vi "SetStart_popup.vi"(0 "Input Line Command":string, 3 "error in (no error)":errorcluster, 5 "Delta Trigger":string, 7 "Trigger":string) -> (8 "Output Line Command":string, 9 "Cancel":bool, 10 "error out":errorcluster)   [LabVIEW 2019]
panel:
  in  "platform":u16(ring) items=["Mac", "PC"]
  in  "Cancel button":bool
  in  "OK Button":bool
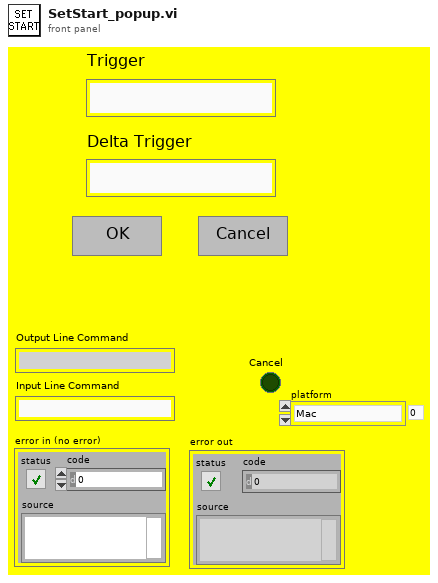
[diagram p1: front panel]
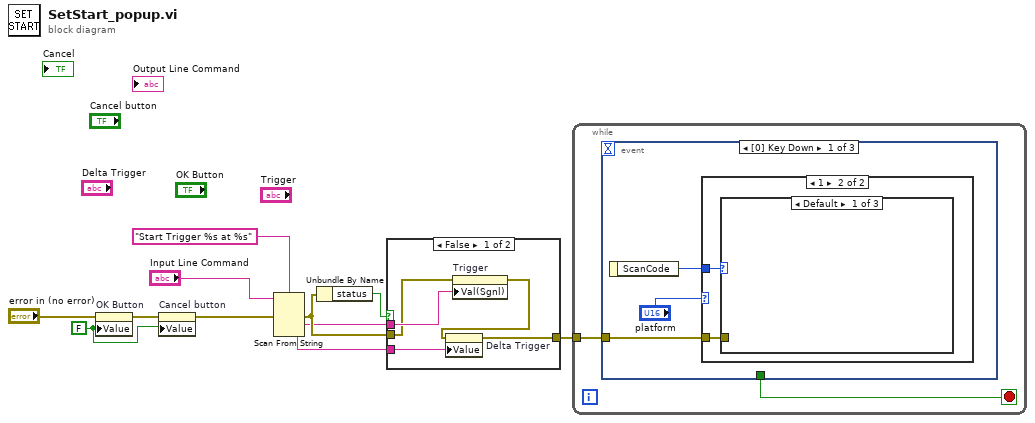
[diagram p0: block diagram]
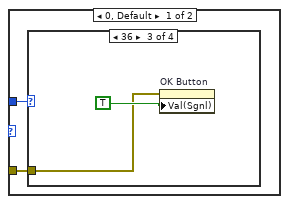
[diagram p2: hidden frame]
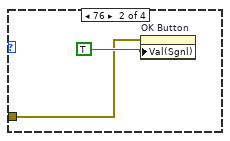
[diagram p4: hidden frame]
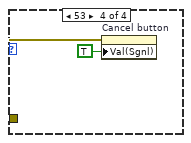
[diagram p5: hidden frame]
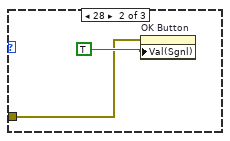
[diagram p6: hidden frame]
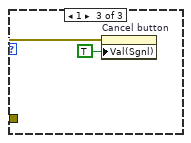
[diagram p7: hidden frame]
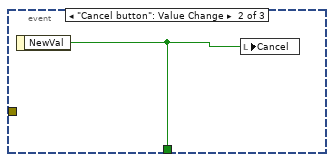
[diagram p8: hidden frame]
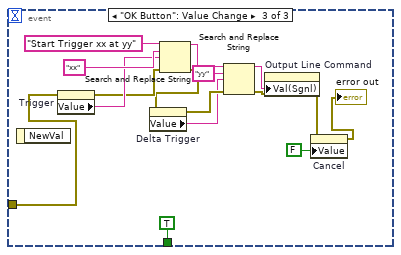
[diagram p9: hidden frame]
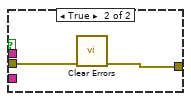
[diagram p10: hidden frame]
diagram:
  w11 = FALSE ("OK Button")
  n1 = property on="OK Button" class="Bool (strict)"(error in="error in (no error)", "Value"=w11) -> (error out=w10:errorcluster)  [unwired: 1 in, 1 out]
  n2 = property on="Cancel button" class="Bool (strict)"(error in=w10, "Value"=w11) -> (error out=w8:errorcluster)  [unwired: 1 in, 1 out]
  n3 = Scan From String(format string="Start Trigger %s at %s", input string="Input Line Command", error in=w8) -> (error out=w5:errorcluster, output 1=w4:string, output 2=w3:string)  [unwired: 3 in, 2 out]
  n4 = Unbundle By Name(w5) -> ("status"=w6:bool)
  n5 = case shown="False" w6 {
    tunnel: w5 -> [w14 w18]
    tunnel: w4 -> [w16 _]
    tunnel: w3 -> [w15 _]
    tunnel: [w12 w17] -> w1
    frame False {
      n6 = property on="Trigger" class="Str"(error in=w14, "Val(Sgnl)"=w16) -> (error out=w13:errorcluster)  [unwired: 1 in, 1 out]
      n7 = property on="Delta Trigger" class="Str"(error in=w13, "Value"=w15) -> (error out=w12:errorcluster)  [unwired: 1 in, 1 out]
    }
    frame True {
      n8 = call <vilib>:"Clear Errors.vi"("error in (no error)"=w18) -> ("error out"=w17:errorcluster)  [unwired: 5 in, 1 out]
    }
  }
  n9 = while {
    tunnel: w1 -> [w20]
    stop <- w19 stop-if-true
    n10 = event shown="[0] Key Down" {
      selector: _ -> [_ _ _]
      dyn-events: _ -> [_ _ _]
      timeout: _ -> [_ _ _]
      tunnel: w20 -> [w23 _ w51]
      tunnel: [_ w38 TRUE ("NewVal")] -> w19
      event Key Down {
        n11 = event-data() -> ("ScanCode"=w22:i16)  [unwired: 1 in]
        n12 = case shown="1" "platform" {
          tunnel: w23 -> [w25 w33]
          tunnel: w22 -> [w24 w32]
          frame 0, Default {
            n13 = case shown="36" w24 {
              tunnel: w25 -> [_ w26 w28 w30]
              frame Default {
              }
              frame 76 {
                n14 = property on="OK Button" class="Bool (strict)"(error in=w26, "Val(Sgnl)"=TRUE ("Value (Signaling)")) -> ()  [unwired: 1 in, 2 out]
              }
              frame 36 {
                n15 = property on="OK Button" class="Bool (strict)"(error in=w28, "Val(Sgnl)"=TRUE ("Value (Signaling)")) -> ()  [unwired: 1 in, 2 out]
              }
              frame 53 {
                n16 = property on="Cancel button" class="Bool (strict)"(error in=w30, "Val(Sgnl)"=TRUE ("Value (Signaling)")) -> ()  [unwired: 1 in, 2 out]
              }
            }
          }
          frame 1 {
            n17 = case shown="Default" w32 {
              tunnel: w33 -> [_ w34 w36]
              frame Default {
              }
              frame 28 {
                n18 = property on="OK Button" class="Bool (strict)"(error in=w34, "Val(Sgnl)"=TRUE ("Value (Signaling)")) -> ()  [unwired: 1 in, 2 out]
              }
              frame 1 {
                n19 = property on="Cancel button" class="Bool (strict)"(error in=w36, "Val(Sgnl)"=TRUE ("Value (Signaling)")) -> ()  [unwired: 1 in, 2 out]
              }
            }
          }
        }
      }
      event "Cancel button": Value Change {
        n20 = event-data() -> ("NewVal"=w38:bool)  [unwired: 1 in]
        n21 = local write "Cancel"(w38) -> ()
      }
      event "OK Button": Value Change {
        n22 = event-data() -> ()  [unwired: 1 in, 1 out]
        n23 = property on="Trigger" class="Str"(error in=w51) -> (error out=w50:errorcluster, "Value"=w52:string)  [unwired: 1 in, 1 out]
        n24 = Search and Replace String(input string="Start Trigger xx at yy" ("format string"), search string="xx", replace string=w52, error in=w50) -> (result string=w49:string, error out=w47:errorcluster)  [unwired: 4 in, 2 out]
        n25 = property on="Delta Trigger" class="Str"(error in=w47) -> (error out=w46:errorcluster, "Value"=w45:string)  [unwired: 1 in, 1 out]
        n26 = Search and Replace String(input string=w49, search string="yy", replace string=w45, error in=w46) -> (result string=w44:string, error out=w43:errorcluster)  [unwired: 4 in, 2 out]
        n27 = property on="Output Line Command" class="Str"(error in=w43, "Val(Sgnl)"=w44) -> (error out=w41:errorcluster)  [unwired: 1 in, 1 out]
        n28 = property on="Cancel" class="Bool (strict)"(error in=w41, "Value"=FALSE ("Cancel")) -> (error out=→"error out":errorcluster)  [unwired: 1 in, 1 out]
      }
    }
  }
